vi "CPP_Aeroprobe-MultiProbeQuickSpare.vi"() -> (5 "Plug in titles":string[](array[string]), 7 "Plug in values":string[](array[string]))   [LabVIEW 2013]
uses:
  Globals/Meas_global.vi
panel:
  in  "Old5HoleProbe?":bool
  out "return type":i32
  out "p-p0":dbl[](array[numeric]) format="%#.5f"
  out "Temperature/C":dbl format="%#.1f"
  out "Pressure/mBar":dbl
  out "timeOfzero":timestamp
  out "zeroShift/mmH2O":dbl[](array[numeric]) format="%#.6f"
  in  "Mode":enum32{"Measure", "Take Zeroes"}(radio)=enum."Take Zeroes"
  out "Velocity":dbl
  out "W":dbl
  out "V":dbl
  out "U":dbl caption="u  m/s"
  # "!!     5-hole 1-5 must be connected to Channels 1-5       !!\n!! Old 5-hole on 9- 13;  use this VI if reducing 2 probes !!"
  # "Zero Info"
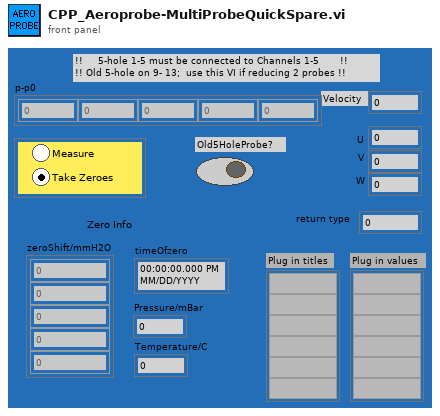
[diagram p1: front panel]
types:
  T1 = typedef "Analysis_info_cluster.ctl" = cluster{"Colour":u32, "Inst type":T2, "Inst name":string, "Symbol":string, "Code name":string, "Extra Info":string, "Inst Array":T3, "Extra Titles":string[], "Extra Values":string[], "U":dbl, "u^2":dbl, "u^3":dbl, "u^4":dbl, "Skew_u":dbl, "Kurt_u":dbl, "Sd Error in Mean":dbl, "% u'/U":dbl, "X":dbl, "Y":dbl, "Z":dbl, "Timescale integral to 25%":dbl, "Sd Error in Variance":dbl, "Calib File":path, "Calib Constants":dbl[], "Output Position":bool, "Full Stats":bool, "Av Sampling Rate":dbl, "Av No of Samples":dbl, "Total Meas Time (s)":dbl, "ADAM Ch Name":string}
  T2 = typedef "Inst_type.ctl" = enum16{"Propeller anemometer", "Raw voltage", "Pressure Transducer", "Pitot-static tube", "Preston tube", "Hot wire", "Cross wire 1", "Cross wire 2", "Generic Linear", "Generic Polynomial", "Generic BackPoly", "Fast FID", "Thermocouple", "Cold wire", "Pulsed Wire", "LDA Vel", "LDA Tran time", "LDA Arr time"}
  T3 = typedef "Instrument_Array.ctl" = enum16{"PWA", "LDA", "Analogue"}
  T4 = cluster{"Analysis Info cluster[0]":T1, "Analysis Info cluster[1]":T1, "Analysis Info cluster[2]":T1, "Analysis Info cluster[3]":T1, "Analysis Info cluster[4]":T1, "Analysis Info cluster[5]":T1, "Analysis Info cluster[6]":T1}
  T5 = cluster{"Analysis Info cluster[0]":T1, "Analysis Info cluster[1]":T1, "Analysis Info cluster[2]":T1, "Analysis Info cluster[3]":T1, "Analysis Info cluster[4]":T1, "Analysis Info cluster[5]":T1, "Analysis Info cluster[6]":T1, "Analysis Info cluster[7]":T1, "Analysis Info cluster[8]":T1, "Analysis Info cluster[9]":T1, "Analysis Info cluster[10]":T1, "Analysis Info cluster[11]":T1, "Analysis Info cluster[12]":T1, "Analysis Info cluster[13]":T1}
  T6 = cluster{"[0]":dbl, "[1]":dbl, "[2]":dbl, "[3]":dbl, "[4]":dbl}
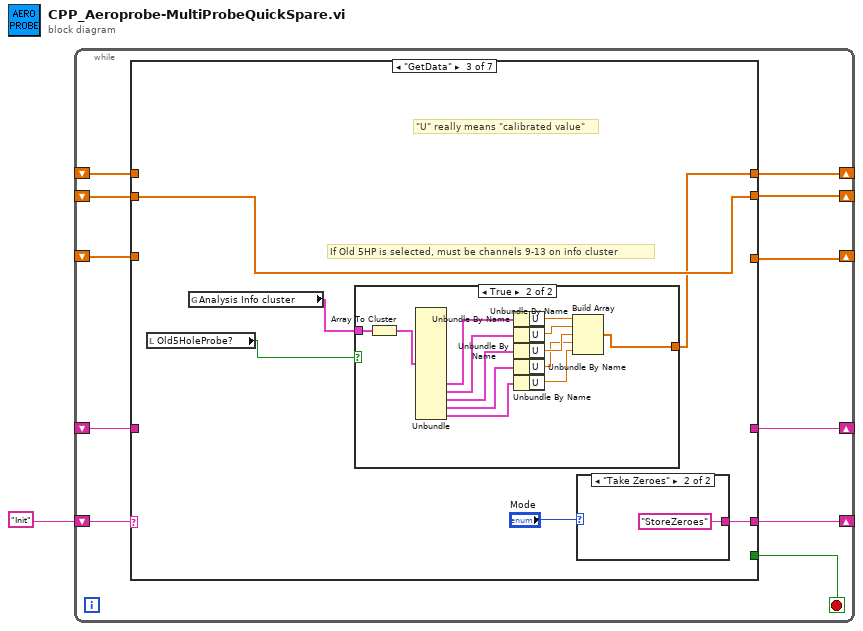
[diagram p0: block diagram]
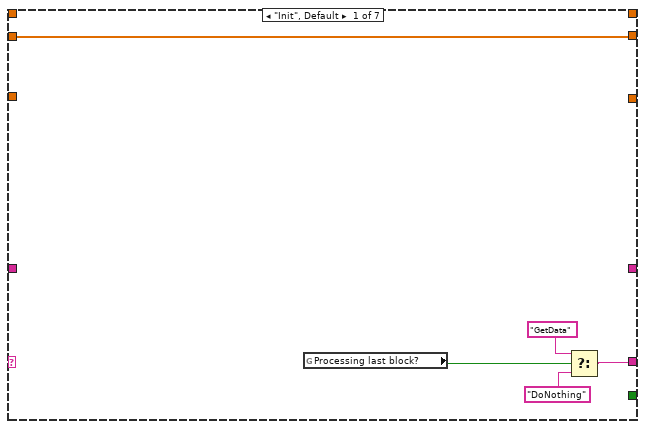
[diagram p2: hidden frame]
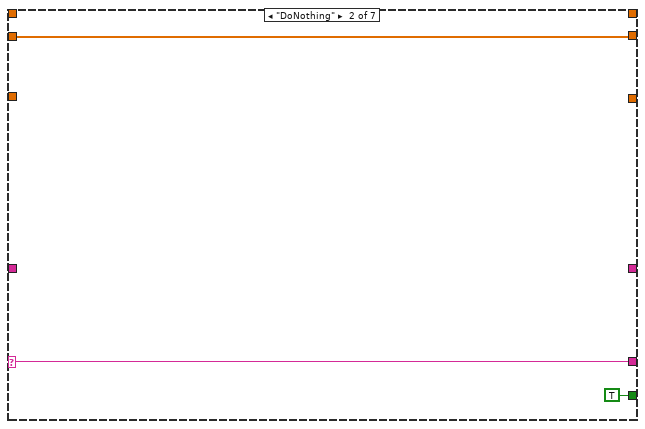
[diagram p3: hidden frame]
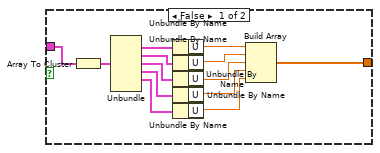
[diagram p4: hidden frame]
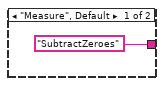
[diagram p5: hidden frame]
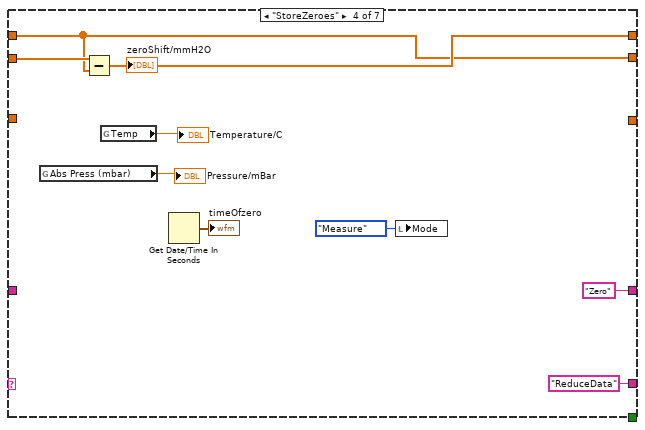
[diagram p6: hidden frame]
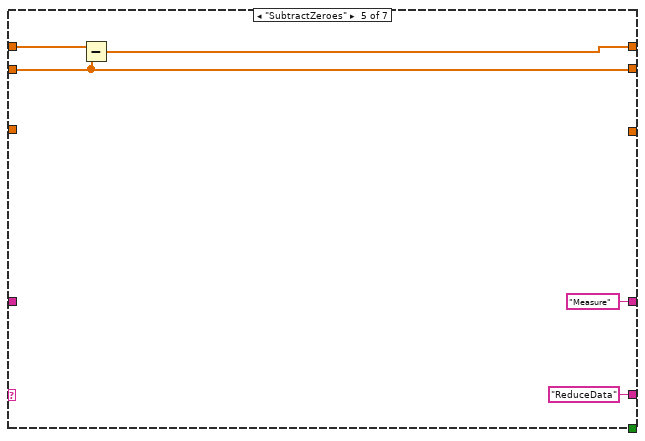
[diagram p7: hidden frame]
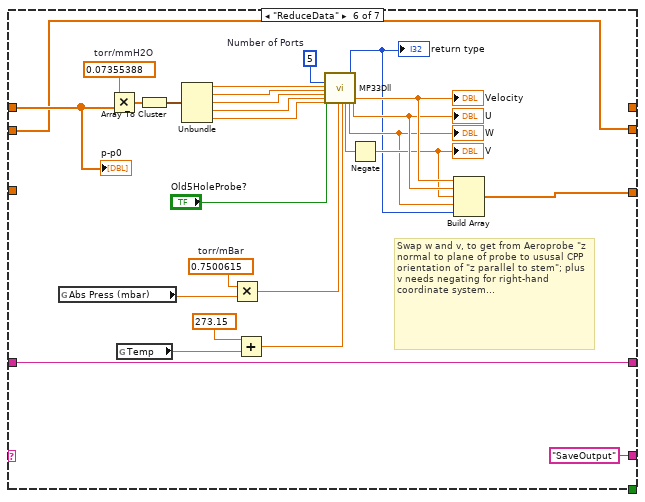
[diagram p8: hidden frame]
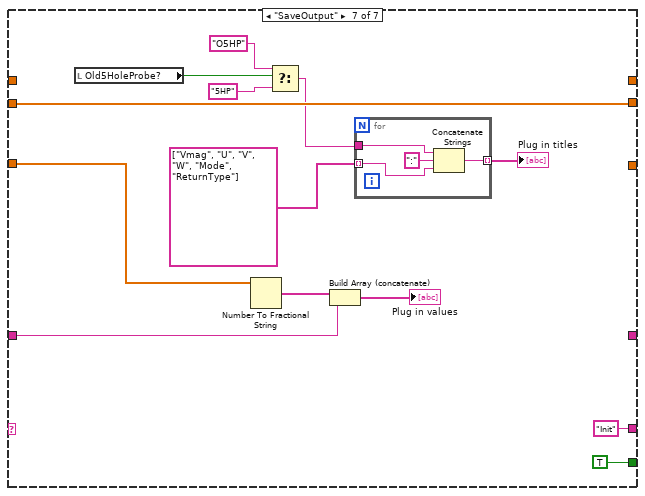
[diagram p9: hidden frame]
diagram:
  n1 = while {
    shift-right: [w11] -> _
    shift-left: "Init" -> [w12]
    shift-right: [w10] -> _
    shift-left: _ -> [w8]
    shift-right: [w9] -> _
    shift-left: _ -> [w7]
    shift-right: [w6] -> _
    shift-left: _ -> [w5]
    shift-right: [w3] -> _
    shift-left: _ -> [w2]
    stop <- w4 stop-if-true
    n2 = case shown="\"GetData\"" w12 {
      selector: w12 -> [_ w20 _ _ _ _ _]
      tunnel: [w17 w20 w26 "ReduceData" "ReduceData" "SaveOutput" "Init"] -> w11
      tunnel: [_ _ w21 w61 w67 _ _] -> w10
      tunnel: [w13 w18 w24 w55 w66 w80 w108] -> w9
      tunnel: w8 -> [_ _ _ w55 w68 w89 _]
      tunnel: w7 -> [w13 w18 w24 w63 w66 w80 w108]
      tunnel: [_ _ _ _ _ w76 _] -> w6
      tunnel: w5 -> [_ _ _ _ _ _ w107]
      tunnel: [_ TRUE _ _ _ _ TRUE] -> w4
      tunnel: [_ _ _ "Zero" "Measure" w75 _] -> w3
      tunnel: w2 -> [_ _ _ _ _ w75 w102]
      frame "Init", Default {
        n3 = global read "Meas_global.vi" "Processing last block?"() -> (w16:bool)
        n4 = Select(t="GetData", s=w16, f="DoNothing") -> (s? t:f=w17:string)
      }
      frame "DoNothing" {
      }
      frame "GetData" {
        # "If Old 5HP is selected, must be channels 9-13 on info cluster"
        # "\"U\" really means \"calibrated value\""
        n5 = local read "Old5HoleProbe?"() -> (w23:bool)
        n6 = global read "Meas_global.vi" "Analysis Info cluster"() -> (w22:T1[])
        n7 = case shown="True" w23 {
          tunnel: w22 -> [w28 w48]
          tunnel: [w27 w42] -> w21
          frame False {
            n8 = Array To Cluster(array=w28) -> (cluster=w34:T4)
            n9 = Unbundle(w34) -> ("Analysis Info cluster[1]"=w33:T1, "Analysis Info cluster[2]"=w32:T1, "Analysis Info cluster[3]"=w31:T1, "Analysis Info cluster[4]"=w30:T1, "Analysis Info cluster[5]"=w29:T1)  [unwired: 2 out]
            n10 = Unbundle By Name(w33) -> ("U"=w35:dbl)
            n11 = Unbundle By Name(w32) -> ("U"=w36:dbl)
            n12 = Unbundle By Name(w31) -> ("U"=w37:dbl)
            n13 = Unbundle By Name(w30) -> ("U"=w38:dbl)
            n14 = Unbundle By Name(w29) -> ("U"=w39:dbl)
            n15 = Build Array(w35, w36, w37, w38, w39) -> (w27:dbl[])
          }
          frame True {
            n16 = Array To Cluster(array=w48) -> (cluster=w49:T5)
            n17 = Unbundle(w49) -> ("Analysis Info cluster[9]"=w47:T1, "Analysis Info cluster[10]"=w46:T1, "Analysis Info cluster[11]"=w45:T1, "Analysis Info cluster[12]"=w44:T1, "Analysis Info cluster[13]"=w43:T1)  [unwired: 9 out]
            n18 = Unbundle By Name(w47) -> ("U"=w50:dbl)
            n19 = Unbundle By Name(w46) -> ("U"=w51:dbl)
            n20 = Unbundle By Name(w45) -> ("U"=w41:dbl)
            n21 = Unbundle By Name(w44) -> ("U"=w40:dbl)
            n22 = Unbundle By Name(w43) -> ("U"=w52:dbl)
            n23 = Build Array(w50, w51, w41, w40, w52) -> (w42:dbl[])
          }
        }
        n24 = case shown="\"Take Zeroes\"" "Mode" {
          tunnel: ["SubtractZeroes" "StoreZeroes"] -> w26
          frame "Measure", Default {
          }
          frame "Take Zeroes" {
          }
        }
      }
      frame "StoreZeroes" {
        n25 = global read "Meas_global.vi" "Abs Press (mbar)"() -> (→"Pressure/mBar":dbl)
        n26 = Subtract(x=w63, y=w55) -> (x-y=w61:dbl[])
        "zeroShift/mmH2O" <- w61
        n27 = global read "Meas_global.vi" "Temp"() -> (→"Temperature/C":dbl)
        n28 = Get Date/Time In Seconds() -> (seconds since 1Jan1904=→"timeOfzero":timestamp)
        n29 = local write "Mode"(enum32{"Measure", "Take Zeroes"}."Measure" ("Mode")) -> ()
      }
      frame "SubtractZeroes" {
        n30 = Subtract(x=w68, y=w66) -> (x-y=w67:dbl[])
      }
      frame "ReduceData" {
        w90 = 0.07355388  # torr/mmH2O
        w94 = 0.7500615  # torr/mBar
        w91 = 5  # Number of Ports
        # "Swap w and v, to get from Aeroprobe \"z normal to plane of probe to ususal CPP orientation of \"z parallel to stem\"; plus v needs negating for right-hand coordinate system..."
        n31 = global read "Meas_global.vi" "Abs Press (mbar)"() -> (w71:dbl)
        n32 = Multiply(x=w90, y=w89) -> (x*y=w88:dbl[])
        n33 = global read "Meas_global.vi" "Temp"() -> (w72:dbl)
        n34 = Array To Cluster(array=w88) -> (cluster=w87:T6)
        n35 = Unbundle(w87) -> ("[0]"=w86:dbl, "[1]"=w85:dbl, "[2]"=w84:dbl, "[3]"=w83:dbl, "[4]"=w82:dbl)
        n36 = Multiply(x=w94, y=w71) -> (x*y=w93:dbl)
        n37 = Add(x=273.15, y=w72) -> (x+y=w95:dbl)
        n38 = call "MP33Dll.vi"("Old5HoleProbe?"="Old5HoleProbe?", "Number of Ports"=w91, "P1 Torr"=w86, "P2 Torr"=w85, "P3 Torr"=w84, "P4 Torr"=w83, "P5 Torr"=w82, "Pref Torr"=w93, "TTot Kelvin"=w95) -> ("w m/s"=w77:dbl, "return type"=w70:i32, "v m/s"=w73:dbl, "VMagn m/s"=w79:dbl, "u  m/s"=w78:dbl)  [unwired: 8 in, 6 out]
        "U" <- w78
        "W" <- w73
        "Velocity" <- w79
        "return type" <- w70
        n39 = Negate(x=w77) -> (-x=w74:dbl)
        "V" <- w74
        n40 = Build Array(w79, w78, w74, w73, w70) -> (w76:dbl[])
        "p-p0" <- w89
      }
      frame "SaveOutput" {
        n41 = local read "Old5HoleProbe?"() -> (w100:bool)
        n42 = Number To Fractional String(number=w107) -> (F-format string=w106:string[])  [unwired: 3 in]
        n43 = Select(t="O5HP", s=w100, f="5HP") -> (s? t:f=w97:string)
        n44 = Build Array (concatenate)(w106, w102) -> (→"Plug in values":string[])
        n45 = for {
          tunnel: string[] ["Vmag", "U", "V", "W", "Mode", "ReturnType"] ("Plug in titles") -> [w110] mode=indexing
          tunnel: w97 -> [w112]
          tunnel: [w109] -> w96 mode=indexing
          n46 = Concatenate Strings(w112, ":" ("string"), w110) -> (w109:string)
        }
        "Plug in titles" <- w96
      }
    }
  }
